vi "test Connect.vi"(8 "error in (no error)":errorcluster, 11 "TestCase in":refnum<class "Switch Consumer Test Case.lvclass">) -> (0 "error out":errorcluster, 3 "TestCase out":refnum<class "Switch Consumer Test Case.lvclass">)   [LabVIEW 2017, in "Switch Consumer Test Case.lvclass"]
uses:
  Switch Consumer Test Case.lvclass
  Switch/Switch Connect Message/Switch Connect Message.lvclass
  C:/github/niveristand-custom-device-message-library/Source/Message/Abstract Message/Abstract Message.lvclass
  Support/Message String Action.ctl
  Switch Consumer Test Case.lvclass/Switch Consumer Test Case.ctl
  Producer/Abstract Producer/Abstract Producer.lvclass
  <vilib>/addons/_JKI Toolkits/VI Tester/TestCase.llb/TestCase.lvclass
  Consumer/Abstract Consumer/Abstract Consumer.lvclass
  C:/Program Files (x86)/National Instruments/LabVIEW 2017/vi.lib/addons/_JKI Toolkits/VI Tester/TestCase.llb/TestCase.lvclass
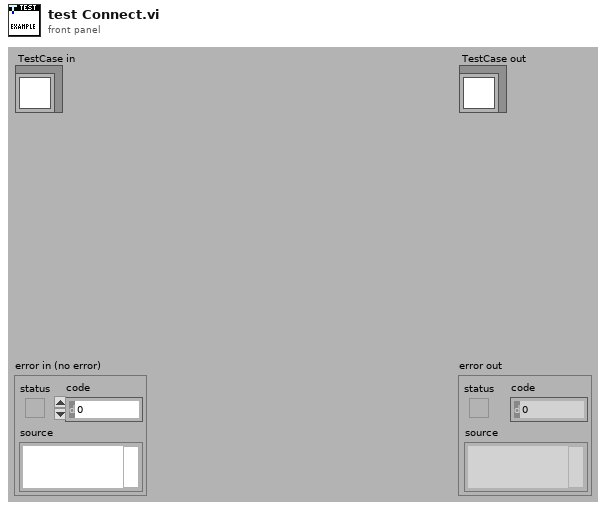
[diagram p1: front panel]
types:
  T1 = typedef "Message String Action.ctl" = enum16{"Get String", "Set String", "Reset"}
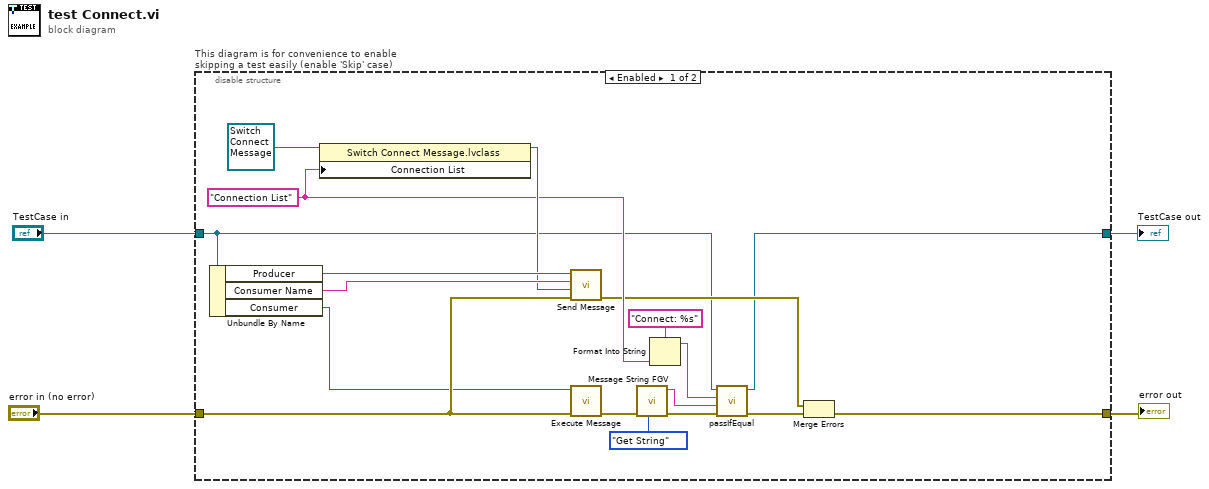
[diagram p0: block diagram]
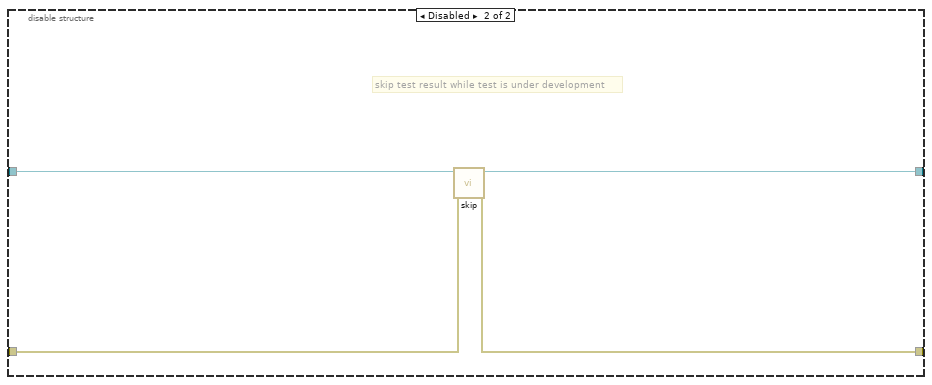
[diagram p2: hidden frame]
diagram:
  n1 = disable-structure "This diagram is for convenience to enable skipping a test easily (enable 'Skip' case)" shown="Enabled" {
    disable-tunnel: "TestCase in" -> [w6 w26]
    disable-tunnel: [w5 w24] -> w1
    disable-tunnel: [w7 w25] -> w3
    disable-tunnel: "error in (no error)" -> [w21 w23]
    frame Enabled {
      w12 = "Connection List"
      n2 = Unbundle By Name(w6) -> ("Producer"=w22:refnum<class "Abstract Producer.lvclass">, "Consumer Name"=w19:string, "Consumer"=w20:refnum<class "Abstract Consumer.lvclass">)
      n3 = property class="Switch Connect Message.lvclass"(reference=refnum<class "Switch Connect Message.lvclass"> refnum ("Messaging.lvlib:Switch.lvlib:Switch Connect Message.lvclass"), "Connection List"=w12) -> (reference out=w17:refnum<class "Switch Connect Message.lvclass">)  [unwired: 1 in, 1 out]
      n4 = call-dynamic "Send Message.vi"("error in (no error)"=w21, "Message in"=w17, "Consumer in"=w19, "Abstract Producer in"=w22) -> ("error out"=w8:errorcluster)  [unwired: 5 in, 2 out]
      n5 = call "Execute Message.vi"("error in (no error)"=w21, "Abstract Consumer in"=w20) -> ("error out"=w15:errorcluster)  [unwired: 7 in, 2 out]
      n6 = call "Message String FGV.vi"("Action"=Message_String_Action."Get String", "error in (no error)"=w15) -> ("error out"=w14:errorcluster, "String out"=w10:string)  [unwired: 8 in]
      n7 = Format Into String(format string="Connect: %s", w12) -> (resulting string=w11:string)  [unwired: 2 in, 1 out]
      n8 = call-dynamic "passIfEqual.vi"("error in (no error)"=w14, "y"=w10, "x"=w11, "TestCase in"=w6) -> ("error out"=w9:errorcluster, "TestCase out"=w5:refnum<class "Switch Consumer Test Case.lvclass">)  [unwired: 6 in]
      n9 = Merge Errors(w8, w9) -> (w7:errorcluster)
    }
    frame Disabled {
      # "skip test result while test is under development"
      n10 = call <vilib>:"skip.vi"("error in (no error)"=w23, "TestCase in"=w26) -> ("error out"=w25:errorcluster, "TestCase out"=w24:refnum<class "Switch Consumer Test Case.lvclass">)  [unwired: 8 in]
    }
  }
  "error out" <- w3
  "TestCase out" <- w1
